vi "Vector Arrow.vi"(0 "Magnitude":dbl=1.0, 1 "Initial Vector":cluster{"Initial":cdb, "Endpoint":cdb}, 5 "Phase, deg":dbl, 9 "Accumulate Phase (F)":bool, 12 "Length, %":dbl=10.0 format="%#_13g", 13 "Offset, deg":dbl=20.0) -> (3 "Resultant Vector":cluster{"Initial":cdb, "Endpoint":cdb}, 4 "XY Graph - Light":cdb[](graph))   [LabVIEW 2025]
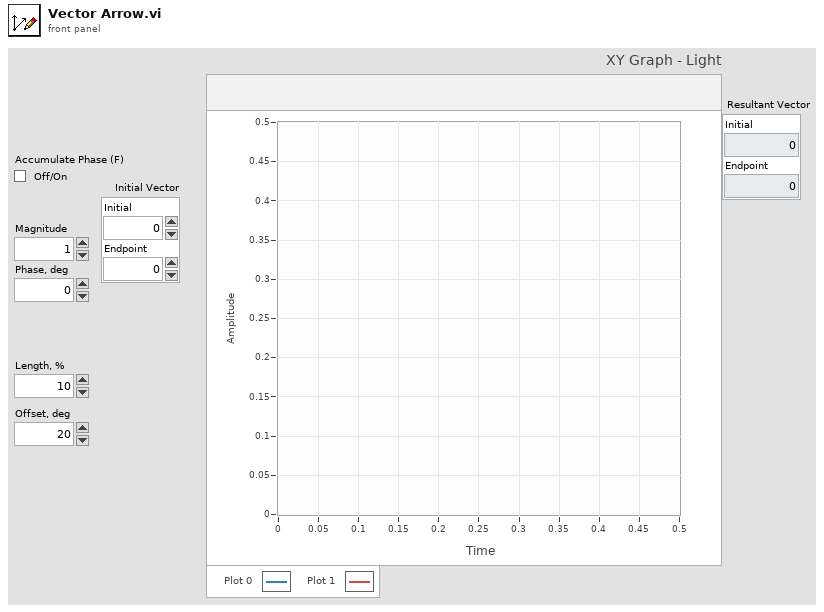
[diagram p1: front panel]
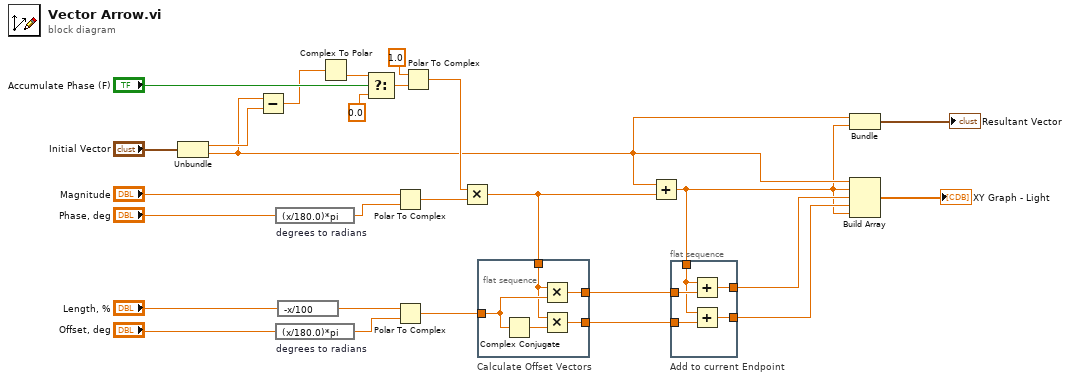
[diagram p0: block diagram]
diagram:
  n1 = Unbundle("Initial Vector") -> ("Initial"=w5:cdb, "Endpoint"=w4:cdb)
  n2 = Subtract(x=w4, y=w5) -> (x-y=w3:cdb)
  n3 = expression code="(x/180.0)*pi" "degrees to radians"("Phase, deg") -> (w12:dbl)
  n4 = expression code="(x/180.0)*pi" "degrees to radians"("Offset, deg") -> (w21:dbl)
  n5 = expression code="-x/100"("Length, %") -> (w17:dbl)
  n6 = Complex To Polar(r * e^(i*theta)=w3) -> (theta=w6:dbl)  [unwired: 1 out]
  n7 = Select(t=w6, s="Accumulate Phase (F)", f=0.0 ("t")) -> (s? t:f=w11:dbl)
  n8 = Polar To Complex(1:w12, 2:"Magnitude") -> (0:w16:cdb)
  n9 = Polar To Complex(1:w21, 2:w17) -> (0:w19:cdb)
  n10 = Polar To Complex(1:w11, 2:1.0 ("t")) -> (0:w9:cdb)
  n11 = Multiply(x=w9, y=w16) -> (x*y=w13:cdb)
  n12 = flat-sequence "Calculate Offset Vectors" {
    tunnel: [w32] -> w27
    tunnel: w19 -> [w31]
    tunnel: w13 -> [w29]
    tunnel: [w28] -> w18
    frame #0 {
      n13 = Complex Conjugate(1:w31) -> (0:w30:cdb)
      n14 = Multiply(x=w29, y=w31) -> (x*y=w32:cdb)
      n15 = Multiply(x=w29, y=w30) -> (x*y=w28:cdb)
    }
  }
  n16 = Add(x=w4, y=w13) -> (x+y=w1:cdb)
  n17 = flat-sequence "Add to current Endpoint" {
    tunnel: w27 -> [w37]
    tunnel: [w36] -> w25
    tunnel: [w35] -> w2
    tunnel: w1 -> [w34]
    tunnel: w18 -> [w33]
    frame #0 {
      n18 = Add(x=w34, y=w37) -> (x+y=w36:cdb)
      n19 = Add(x=w34, y=w33) -> (x+y=w35:cdb)
    }
  }
  n20 = Bundle("Endpoint"=w4, w1) -> (→"Resultant Vector":cluster{"Endpoint":cdb, cdb})  [unwired: 1 in]
  n21 = Build Array(w4, w1, w25, w2, w1) -> (→"XY Graph - Light":cdb[])
